vi "Set Timeout.vi"(8 "error in (no error)":errorcluster, 10 "Timeout ms":i32, 11 "WebsocketStream in":refnum<class "WebsocketStream.lvclass">) -> (0 "error out":errorcluster, 3 "WebsocketStream out":refnum<class "WebsocketStream.lvclass">)   [LabVIEW 2020, in "Stream-Websocket.lvlib" / "WebsocketStream.lvclass"]
uses:
  WebsocketStream.lvclass
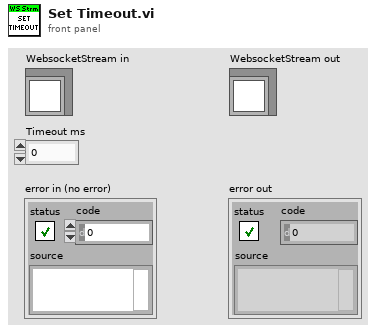
[diagram p1: front panel]
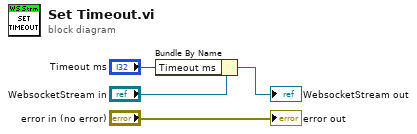
[diagram p0: block diagram]
diagram:
  n1 = Bundle By Name(cluster="WebsocketStream in", "Timeout ms"="Timeout ms") -> (→"WebsocketStream out":refnum<class "WebsocketStream.lvclass">)
  "error out" <- "error in (no error)"
